vi "Unscale and Scale - 16 Bit.vi"(8 "error in (no error)":errorcluster, 11 "Data Scaling in":refnum<class "Data Scaling.lvclass">) -> (0 "error out":errorcluster, 3 "Data Scaling out":refnum<class "Data Scaling.lvclass">)   [LabVIEW 2020, in "Unit Tests.lvlib" / "Data Scaling.lvclass"]
uses:
  Data Scaling.lvclass
  Frames & Messages/TypeDefs/Scaling Information.ctl
  Frames & Messages/Utility/Scale Data.vi
  Frames & Messages/Utility/Unscale Data.vi
  <vilib>/addons/_JKI Toolkits/Caraya/classes/Assert/Assert True.vi
  <vilib>/addons/_JKI Toolkits/Caraya/classes/Test/Test.lvclass
  BCI-1553 API.lvlib
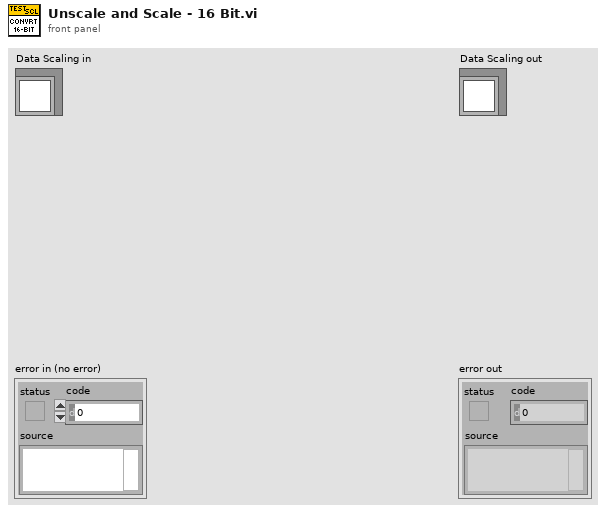
[diagram p1: front panel]
types:
  T1 = typedef "BCI-1553 API.lvlib/Scaling Information.ctl" = cluster{"Bit Offset":i32, "Bit Count":i32, "LSB Resolution":dbl, "2's Complement":bool, "Big Endian":bool, "Sign Bit":bool}
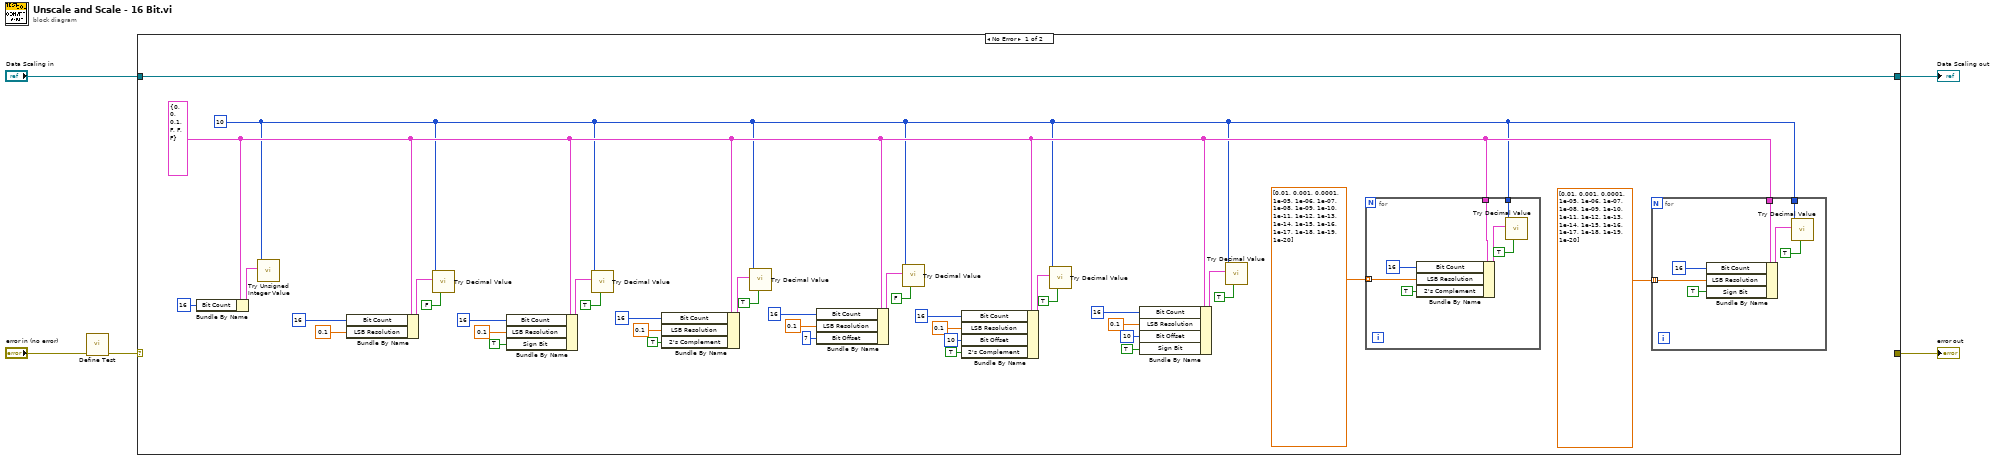
[diagram p0: block diagram]
diagram:
  n1 = call <vilib>:"Define Test.vi"("error in (no error)"="error in (no error)") -> ("error out"=w1:errorcluster)  [unwired: 9 in, 1 out]
  n2 = case shown="No Error" w1 {
    selector: w1 -> [_ w59]
    tunnel: [_ w59] -> w5
    tunnel: [w43 w58] -> w3
    tunnel: "Data Scaling in" -> [w43 w58]
    frame No Error {
      w7 = T1 {"Bit Offset"=0, "Bit Count"=0, "LSB Resolution"=0.1, "2's Complement"=FALSE, "Big Endian"=FALSE, "Sign Bit"=FALSE} ("Scaling Info")
      w6 = 10 ("Random Attempts")
      n3 = Bundle By Name(cluster=w7, "Bit Count"=16) -> (w38:T1)
      n4 = call "Try Unsigned Integer Value.vi"("Scaling Info"=w38, "Random Attempts"=w6) -> ()  [unwired: 9 in, 1 out]
      n5 = Bundle By Name(cluster=w7, "Bit Count"=16, "LSB Resolution"=0.1) -> (w35:T1)
      n6 = call "Try Decimal Value.vi"("Negate?"=FALSE, "Scaling Info"=w35, "Random Attempts"=w6) -> ()  [unwired: 8 in, 1 out]
      n7 = Bundle By Name(cluster=w7, "Bit Count"=16, "LSB Resolution"=0.1, "Sign Bit"=TRUE) -> (w40:T1)
      n8 = call "Try Decimal Value.vi"("Negate?"=TRUE, "Scaling Info"=w40, "Random Attempts"=w6) -> ()  [unwired: 8 in, 1 out]
      n9 = Bundle By Name(cluster=w7, "Bit Count"=16, "LSB Resolution"=0.1, "2's Complement"=TRUE ("Sign Bit")) -> (w10:T1)
      n10 = call "Try Decimal Value.vi"("Negate?"=TRUE, "Scaling Info"=w10, "Random Attempts"=w6) -> ()  [unwired: 8 in, 1 out]
      n11 = Bundle By Name(cluster=w7, "Bit Count"=16, "LSB Resolution"=0.1, "Bit Offset"=7) -> (w31:T1)
      n12 = call "Try Decimal Value.vi"("Negate?"=FALSE, "Scaling Info"=w31, "Random Attempts"=w6) -> ()  [unwired: 8 in, 1 out]
      n13 = Bundle By Name(cluster=w7, "Bit Count"=16, "LSB Resolution"=0.1, "Bit Offset"=10, "2's Complement"=TRUE) -> (w25:T1)
      n14 = call "Try Decimal Value.vi"("Negate?"=TRUE, "Scaling Info"=w25, "Random Attempts"=w6) -> ()  [unwired: 8 in, 1 out]
      n15 = Bundle By Name(cluster=w7, "Bit Count"=16, "LSB Resolution"=0.1, "Bit Offset"=10, "Sign Bit"=TRUE ("2's Complement")) -> (w15:T1)
      n16 = call "Try Decimal Value.vi"("Negate?"=TRUE, "Scaling Info"=w15, "Random Attempts"=w6) -> ()  [unwired: 8 in, 1 out]
      n17 = for {
        tunnel: dbl[] [0.01, 0.001, 0.0001, 1e-05, 1e-06, 1e-07, 1e-08, 1e-09, 1e-10, 1e-11, 1e-12, 1e-13, 1e-14, 1e-15, 1e-16, 1e-17, 1e-18, 1e-19, 1e-20] ("LSB Resolution") -> [w54] mode=indexing
        tunnel: w7 -> [w52]
        tunnel: w6 -> [w51]
        n18 = Bundle By Name(cluster=w52, "Bit Count"=16, "LSB Resolution"=w54, "2's Complement"=TRUE) -> (w57:T1)
        n19 = call "Try Decimal Value.vi"("Negate?"=TRUE, "Scaling Info"=w57, "Random Attempts"=w51) -> ()  [unwired: 8 in, 1 out]
      }
      n20 = for {
        tunnel: dbl[] [0.01, 0.001, 0.0001, 1e-05, 1e-06, 1e-07, 1e-08, 1e-09, 1e-10, 1e-11, 1e-12, 1e-13, 1e-14, 1e-15, 1e-16, 1e-17, 1e-18, 1e-19, 1e-20] ("LSB Resolution") -> [w47] mode=indexing
        tunnel: w7 -> [w45]
        tunnel: w6 -> [w44]
        n21 = Bundle By Name(cluster=w45, "Bit Count"=16, "LSB Resolution"=w47, "Sign Bit"=TRUE ("2's Complement")) -> (w50:T1)
        n22 = call "Try Decimal Value.vi"("Negate?"=TRUE, "Scaling Info"=w50, "Random Attempts"=w44) -> ()  [unwired: 8 in, 1 out]
      }
    }
    frame Error {
    }
  }
  "error out" <- w5
  "Data Scaling out" <- w3
